vi "read_csv_v02.vi"() -> (2 "Step name 给log表头":string[](array[string]), 3 "目标结构体数组":T1(array[cluster]))   [LabVIEW 2024]
uses:
  <vilib>/Utility/file.llb/Read Delimited Spreadsheet (string).vi
panel:
  in  "簇":T2
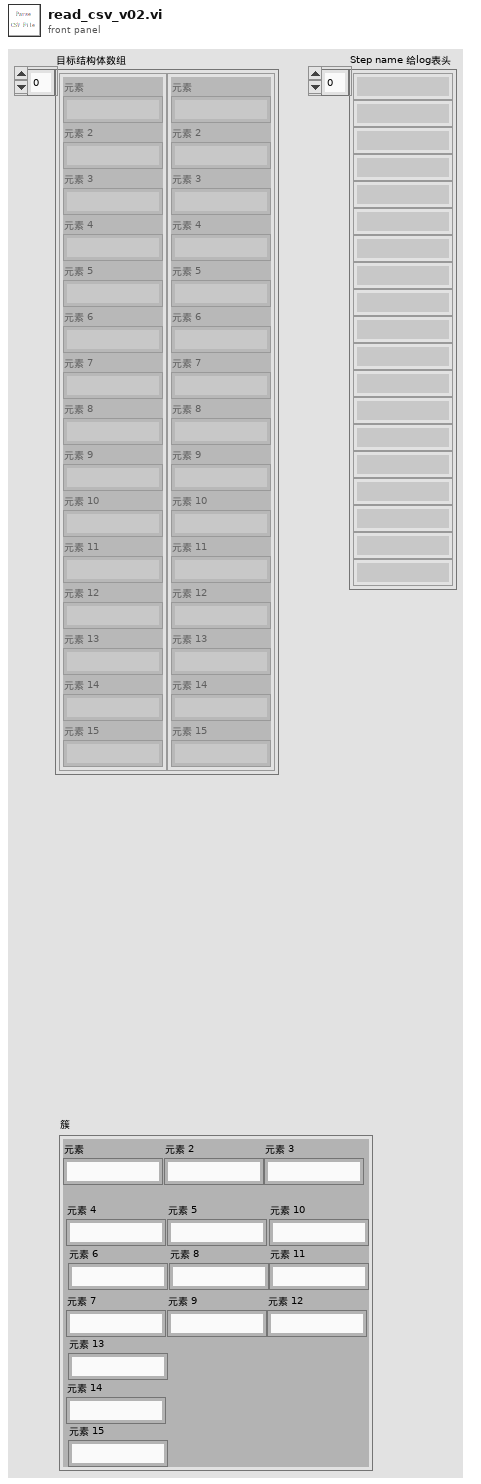
[diagram p1: front panel]
types:
  T1 = cluster{"元素":string, "元素 2":string, "元素 3":string, "元素 4":string, "元素 5":string, "元素 6":string, "元素 7":string, "元素 8":string, "元素 9":string, "元素 10":string, "元素 11":string, "元素 12":string, "元素 13":string, "元素 14":string, "元素 15":string}[]
  T2 = cluster{"元素":string, "元素 2":string, "元素 3":string, "元素 4":string, "元素 5":string, "元素 6":string, "元素 7":string, "元素 8":string, "元素 9":string, "元素 10":string, "元素 11":string, "元素 12":string, "元素 13":string, "元素 14":string, "元素 15":string}
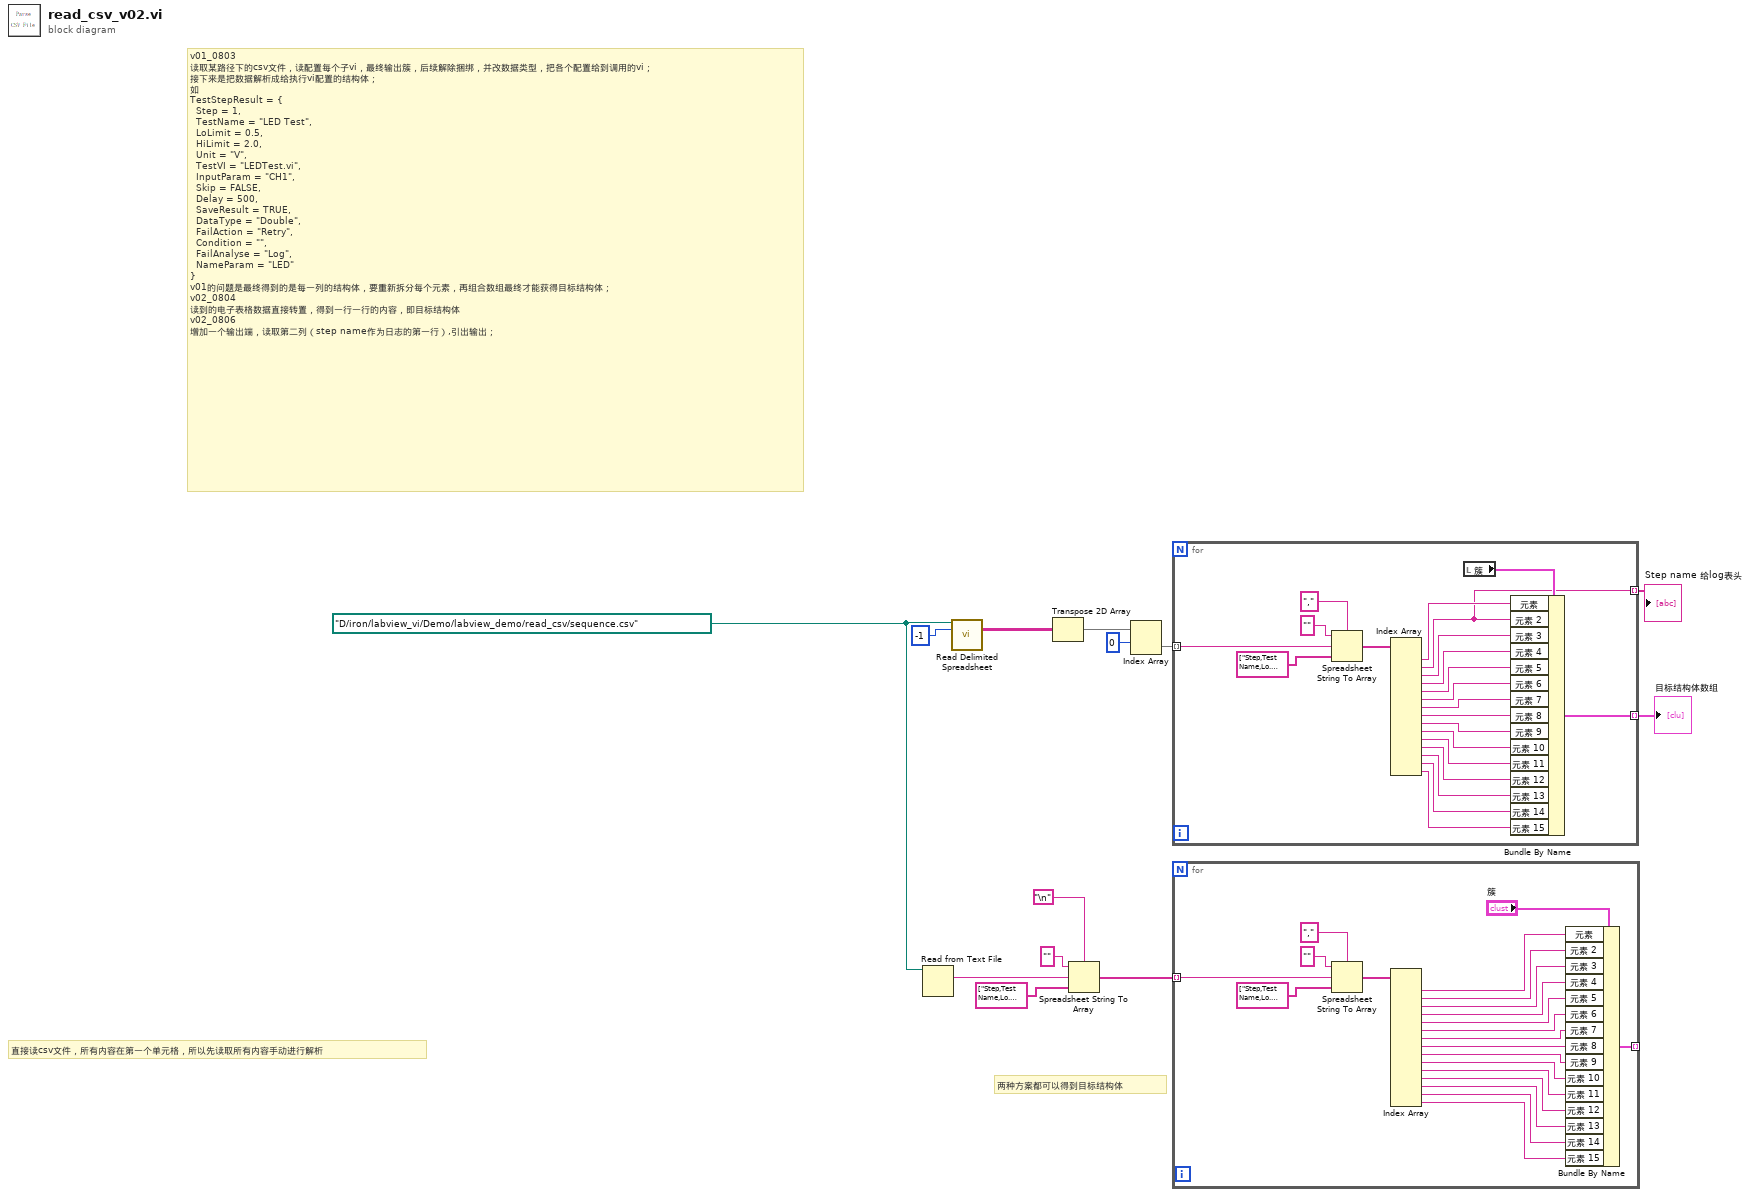
[diagram p0: block diagram]
diagram:
  w12 = path "D:/iron/labview_vi/Demo/labview_demo/read_csv/sequence.csv" ("file path (dialog if empty)")
  # "两种方案都可以得到目标结构体"
  # "直接读csv文件，所有内容在第一个单元格，所以先读取所有内容手动进行解析"
  # "v01_0803\n读取某路径下的csv文件，读配置每个子vi，最终输出簇，后续解除捆绑，并改数据类型，把各个配置给到调用的vi；\n接下来是把数据解析成给执行vi配置的结构体；\n如\nTestStepResult = {\n  Step = 1,\n  TestName = \"LED Test\",\n  LoLimit = 0.5,\n  HiLimit = 2.0,\n  Unit = \"V\",\n  TestVI = \"LEDTest.vi\",\n  InputParam = \"CH1\",\n  Skip = FALSE,\n  Delay = 500,\n  SaveResult = TRUE,\n  DataType = \"Double\",\n  FailAction = \"Retry\",\n  Condition = \"\",\n  FailAnalyse = \"Log\",\n  NameParam = \"LED\"\n}\nv01的问题是最终得到的是每一列的结构体，要重新拆分每个元素，再组合数组最终才能获得目标结构体；\nv02_0804\n读到的电子表格数据直接转置，得到一行一行的内容，即目标结构体\nv02_0806\n增加一个输出端，读取第二列（step name作为日志的第一行）,引出输出；"
  n1 = Read from Text File(file (use dialog)=w12) -> (text=w2:string)  [unwired: 3 in, 3 out]
  n2 = call-poly <vilib>:"Read Delimited Spreadsheet.vi"("file path (dialog if empty)"=w12, "number of rows (all:-1)"=-1) -> ("all rows"=w3:string[][])  [unwired: 8 in, 5 out]
  n3 = Transpose 2D Array(2D array=w3) -> (transposed array=w11:string[][])
  n4 = Spreadsheet String To Array(delimiter (Tab)="\n", format string="" ("格式字符串"), spreadsheet string=w2, array type (2D Dbl)=string[] ["Step,Test Name,Lo.Limit,Hi.Limit,Unit,Test Vi Name,Input Parameter,Skip,Delay,Save Result,Data Type,Fail Action,Condition,Fail Analyse,Name Parameter"] ("添加的数组")) -> (array=w6:string[])
  n5 = Index Array(array=w11, index (row)=0 ("索引 (行)")) -> (element=w9:string[])  [unwired: 1 in]
  n6 = for {
    tunnel: [w32] -> w8 mode=indexing
    tunnel: w9 -> [w16] mode=indexing
    tunnel: [w14] -> w1 mode=indexing
    n7 = Spreadsheet String To Array(delimiter (Tab)="," ("正则表达式"), format string="" ("格式字符串"), spreadsheet string=w16, array type (2D Dbl)=string[] ["Step,Test Name,Lo.Limit,Hi.Limit,Unit,Test Vi Name,Input Parameter,Skip,Delay,Save Result,Data Type,Fail Action,Condition,Fail Analyse,Name Parameter", "1,,,,,,,,,,,,,,", "12,,,,,,,,,,,,,,", ""] ("数组 2")) -> (array=w34:string[])
    n8 = Index Array(array=w34) -> (element #1=w17:string, element #2=w14:string, element #3=w31:string, element #4=w30:string, element #5=w29:string, element #6=w28:string, element #7=w27:string, element #8=w26:string, element #9=w25:string, element #10=w24:string, element #11=w23:string, element #12=w22:string, element #13=w21:string, element #14=w20:string, element #15=w19:string)  [unwired: 15 in]
    n9 = local read "簇"() -> (w15:T2)
    n10 = Bundle By Name(cluster=w15, "元素"=w17, "元素 2"=w14, "元素 3"=w31, "元素 4"=w30, "元素 5"=w29, "元素 6"=w28, "元素 7"=w27, "元素 8"=w26, "元素 9"=w25, "元素 10"=w24, "元素 11"=w23, "元素 12"=w22, "元素 13"=w21, "元素 14"=w20, "元素 15"=w19) -> (w32:T2)
  }
  "目标结构体数组" <- w8
  "Step name 给log表头" <- w1
  n11 = for {
    tunnel: w6 -> [w54] mode=indexing
    tunnel: [w52] -> _ mode=indexing
    n12 = Spreadsheet String To Array(delimiter (Tab)="," ("正则表达式"), format string="" ("格式字符串"), spreadsheet string=w54, array type (2D Dbl)=string[] ["Step,Test Name,Lo.Limit,Hi.Limit,Unit,Test Vi Name,Input Parameter,Skip,Delay,Save Result,Data Type,Fail Action,Condition,Fail Analyse,Name Parameter", "1,,,,,,,,,,,,,,", "12,,,,,,,,,,,,,,", ""] ("数组 2")) -> (array=w56:string[])
    n13 = Index Array(array=w56) -> (element #1=w36:string, element #2=w53:string, element #3=w51:string, element #4=w50:string, element #5=w49:string, element #6=w48:string, element #7=w47:string, element #8=w46:string, element #9=w45:string, element #10=w44:string, element #11=w43:string, element #12=w42:string, element #13=w41:string, element #14=w40:string, element #15=w39:string)  [unwired: 15 in]
    n14 = Bundle By Name(cluster="簇", "元素"=w36, "元素 2"=w53, "元素 3"=w51, "元素 4"=w50, "元素 5"=w49, "元素 6"=w48, "元素 7"=w47, "元素 8"=w46, "元素 9"=w45, "元素 10"=w44, "元素 11"=w43, "元素 12"=w42, "元素 13"=w41, "元素 14"=w40, "元素 15"=w39) -> (w52:T2)
  }
